vi "check if ball hit padle (SubVI).vi"(7 "?":T1=enum."Right Wall", 8 "Nowa pozycja paletki":i32, 9 "Array":bool[](array[boolean]), 10 "lokacja y":i32, 11 "lokacja x":i32) -> (3 "Czy pilka uderzyla w paletke?":bool)   [LabVIEW 2018]
uses:
  right or left wall.ctl
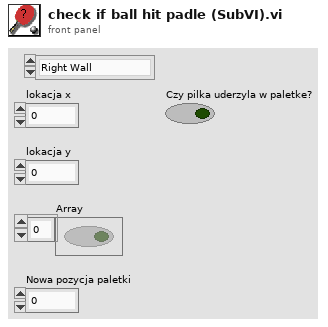
[diagram p1: front panel]
types:
  T1 = typedef "right or left wall.ctl" = enum16{"Left Wall", "Right Wall"}
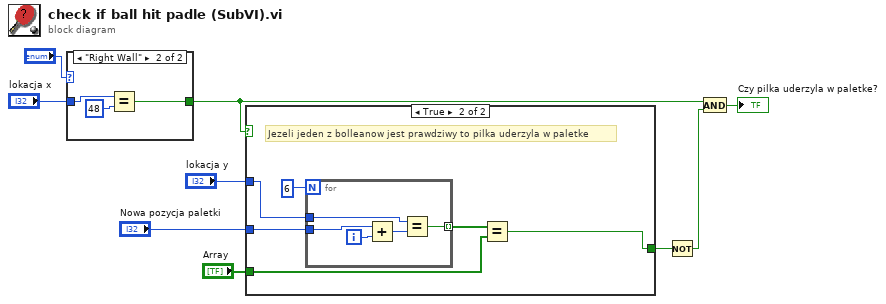
[diagram p0: block diagram]
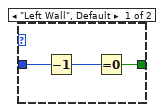
[diagram p2: hidden frame]
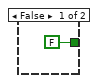
[diagram p3: hidden frame]
diagram:
  n1 = case shown="\"Right Wall\"" "?" {
    tunnel: "lokacja x" -> [w12 w15]
    tunnel: [w10 w13] -> w2
    frame "Left Wall", Default {
      n2 = Decrement(x=w12) -> (x-1=w11:i32)
      n3 = Equal To 0?(x=w11) -> (x = 0?=w10:bool)
    }
    frame "Right Wall" {
      n4 = Equal?(x=w15, y=48) -> (x = y?=w13:bool)
    }
  }
  n5 = case shown="True" w2 {
    tunnel: "lokacja y" -> [_ w21]
    tunnel: "Nowa pozycja paletki" -> [_ w20]
    tunnel: [FALSE w18] -> w9
    tunnel: "Array" -> [_ w17]
    frame False {
    }
    frame True {
      # "Jezeli jeden z bolleanow jest prawdziwy to pilka uderzyla w paletke"
      n6 = for {
        N: 6 -> [_]
        tunnel: w21 -> [w27]
        tunnel: w20 -> [w23]
        tunnel: [w26] -> w19 mode=indexing
        i -> [w25]
        n7 = Add(x=w23, y=w25) -> (x+y=w24:i32)
        n8 = Equal?(x=w27, y=w24) -> (x = y?=w26:bool)
      }
      n9 = Equal?(x=w19, y=w17) -> (x = y?=w18:bool)
    }
  }
  n10 = Not(x=w9) -> (.not. x?=w5:bool)
  n11 = And(x=w2, y=w5) -> (x .and. y?=→"Czy pilka uderzyla w paletke?":bool)
